vi "Eth Status Read set status.vi"(7 "Status Reference":T1, 8 "error in (no error)":errorcluster, 11 "N":i32) -> (0 "error out":errorcluster, 1 "set state":refnum<queue>)   [LabVIEW 2021, in "Eth Status.lvlib"]
uses:
  Eth Status.lvlib
  Ctl/Status.ctl
  MB_TCP2/MB_TCP_State.ctl
  MB_TCP2/MB_TCP.lvclass
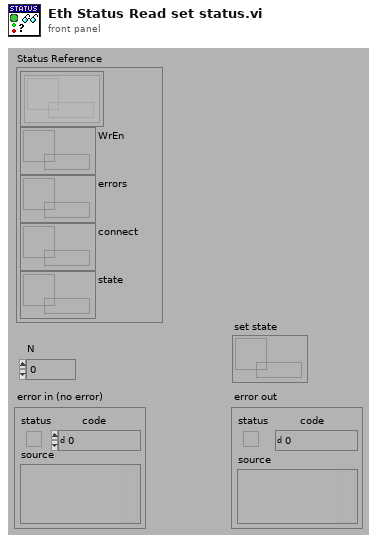
[diagram p1: front panel]
types:
  T1 = typedef "Eth Status.lvlib/Status.ctl" = cluster{"Set_states":refnum<queue>[], "WrEn":refnum<data-value>, "errors":refnum<data-value>, "connect":refnum<data-value>, "state":refnum<data-value>}
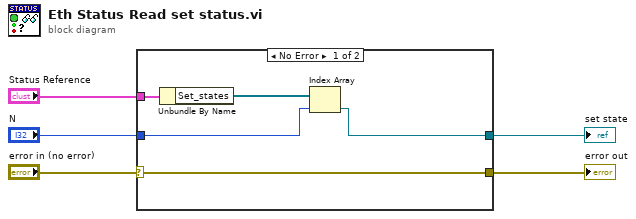
[diagram p0: block diagram]
diagram:
  n1 = case shown="No Error" "error in (no error)" {
    selector: "error in (no error)" -> [w6 w11]
    tunnel: [w6 w11] -> w2
    tunnel: [w10 _] -> w1
    tunnel: "N" -> [w9 _]
    tunnel: "Status Reference" -> [w8 _]
    frame No Error {
      n2 = Unbundle By Name(w8) -> ("Set_states"=w7:refnum<queue>[])
      n3 = Index Array(array=w7, index=w9) -> (element=w10:refnum<queue>)
    }
    frame Error {
    }
  }
  "error out" <- w2
  "set state" <- w1
